vi "modes.vi"() -> ()   [LabVIEW 2019]
panel:
  in  "Array 2":dbl[][](array[numeric])
  out "return value 2":dbl[][](array[numeric])
  out "error out":errorcluster
  in  "return value 3":cluster{"Array 3[0]":dbl, "Array 3[1]":dbl}
  out "return value":cluster{"Array 3[0]":dbl, "Array 3[1]":dbl}
  in  "Array 3":dbl[](array[numeric])
  in  "Array":dbl[](array[numeric])
  in  "Python version":string="3.6"
  in  "function name":string="modes_from_1d_array"
  in  "module path":path=path "C:/Users/edwar/OneDrive/Documents/GitHub/Python-HG-Modes/HG Modes/PauLisa.py"
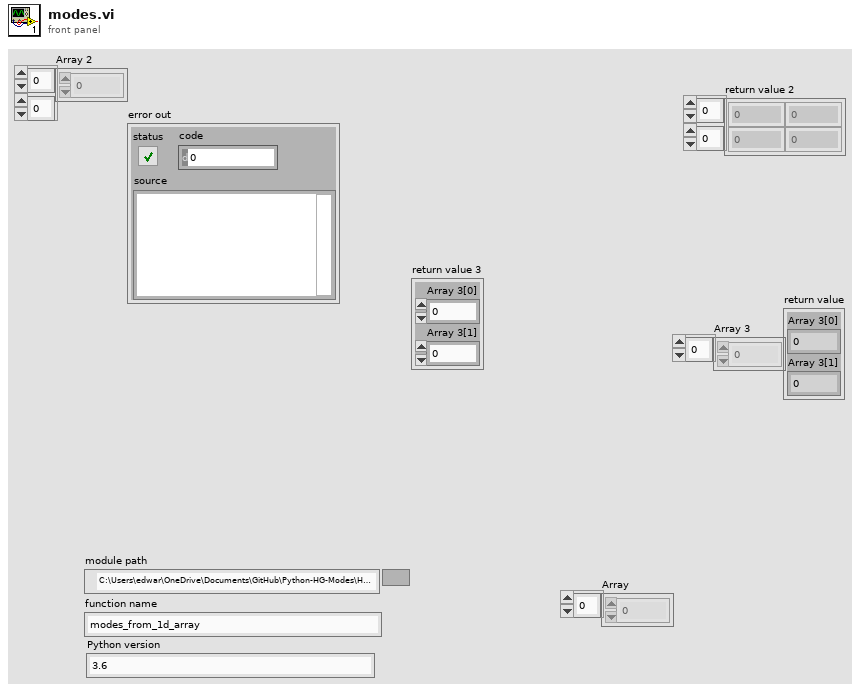
[diagram p1: front panel]
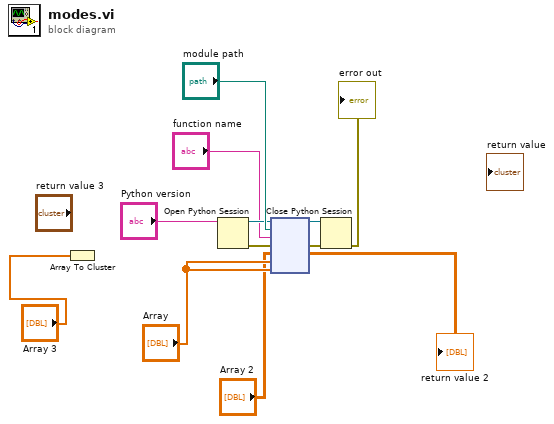
[diagram p0: block diagram]
diagram:
  n1 = Array To Cluster(array="Array 3") -> ()  [unwired: 1 out]
  n2 = Open Python Session(python version="Python version") -> (session out=w10:refnum<k35>, error out=w7:errorcluster)  [unwired: 2 in]
  n3 = node(w10, "module path", "function name", w7, "Array 2", "Array", "Array") -> (w9:refnum<k35>, w6:errorcluster, →"return value 2":dbl[][])  [unwired: 2 in, 2 out]
  "error out" <- w6
  n4 = Close Python Session(session in=w9, error in=w6) -> ()  [unwired: 1 out]
